vi "is image ready for update.vi"(9 "Last update":u32, 10 "min time between updates":u32, 11 "image ref in":T1) -> (3 "update image":bool)   [LabVIEW 2020]
uses:
  <vilib>/vision/Image Controls.llb/IMAQ Image.ctl
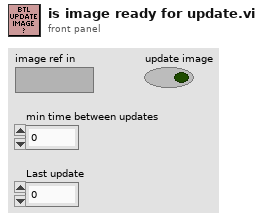
[diagram p1: front panel]
types:
  T1 = typedef "IMAQ Image.ctl" = refnum<image>
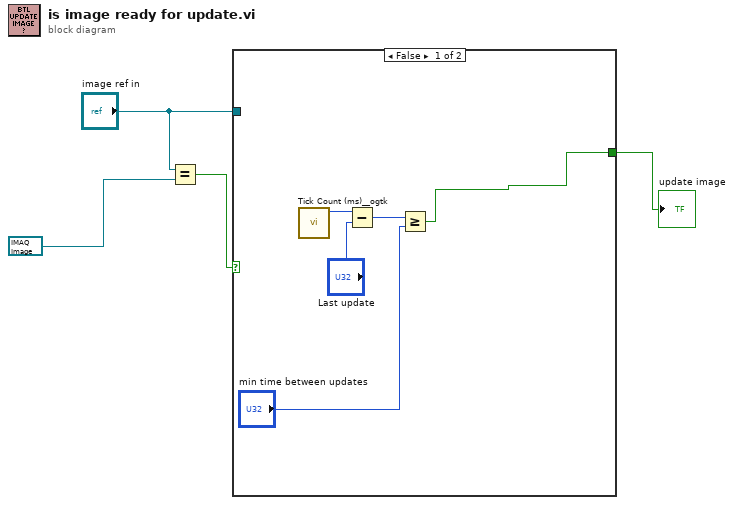
[diagram p0: block diagram]
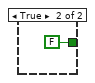
[diagram p2: hidden frame]
diagram:
  n1 = Equal?(x="image ref in", y=T1 refnum ("image ref in 2")) -> (x = y?=w2:bool)
  n2 = case shown="False" w2 {
    tunnel: "image ref in" -> [_ _]
    tunnel: [w5 FALSE] -> w1
    frame False {
      n3 = call <userlib>:"Tick Count (ms)__ogtk.vi"() -> ("millisecond timer value"=w8:u32)  [unwired: 10 in, 1 out]
      n4 = Subtract(x=w8, y="Last update") -> (x-y=w7:u32)
      n5 = Greater Or Equal?(x=w7, y="min time between updates") -> (x >= y?=w5:bool)
    }
    frame True {
    }
  }
  "update image" <- w1
